vi "Transcriptor LabVIEW to C code Arduino Frontend 2.vi"(11 "vi path":path=path "C:/Users/lubo/Documents/LabView/LabVIEW-Universal-Transcriptor/Test/Examples For Parsing/Blink 4 experimental.vi") -> (3 "transcripted code":string="#include <StandardCplusplus.h>\r\n#include <vector>\r\n#include \"ArduinoBasicFunctions.h\"\nusing namespace std;\r\nstruct UserDefined_StructType{String LuboString;\r\nint NumInsideUserCluter;\r\ndouble Double_insideCluster;\r\n};\r\n\r\n\r\n\nvector<bool> Blink_3_simple_and_correct_one(){\n    UserDefined_StructType totoSomNapisalLenTakSVK wireUID_813_ = {\"LuboJe King\",0,0.000000};\r\n    vector<bool> wireUID_770_;\r\n    vector<bool> wireUID_675_ = {true,true,false};\r\n    /***** BEGIN WhileLoop ********/\n    bool wireUID_529_; //LoopEndRef.Wire\n    do{\n        UserDefined_StructType totoSomNapisalLenTakSVK wireUID_682_ = wireUID_813_;\r\n        UserDefined_StructType totoSomNapisalLenTakSVK wireUID_634_;\r\n        vector<bool> wireUID_729_ = wireUID_675_;\r\n        vector<bool> wireUID_701_;\r\n        int wireUID_426_ = 42;\r\n        double wireUID_569_ = 7.000000;\r\n        int wireUID_540_;\r\n        Delay(wireUID_426_); /* by Translator.vi, VI Path: C:\\Users\\lubo\\Documents\\LabView\\LabVIEW-Universal-Transcriptor\\Test\\Examples For Parsing\\Delay.vi */\r\n        wireUID_529_ = wireUID_569_ > wireUID_540_;\r\n        /***** BEGIN CaseStructure ********/\n        \r\n        UserDefined_StructType totoSomNapisalLenTakSVK wireUID_828_ = wireUID_682_;\r\n        vector<bool> wireUID_820_ = wireUID_729_;\r\n        int wireUID_575_ = -42;\r\n        \r\n        UserDefined_StructType totoSomNapisalLenTakSVK wireUID_670_ = wireUID_682_;\r\n        vector<bool> wireUID_720_ = wireUID_729_;\r\n        int wireUID_953_ = -99; //wires declarations\n        switch(wireUID_529_){\n            case false:\n                \r\n                Delay(wireUID_575_); /* by Translator.vi, VI Path: C:\\Users\\lubo\\Documents\\LabView\\LabVIEW-Universal-Transcriptor\\Test\\Examples For Parsing\\Delay.vi */ /* C code */\n                wireUID_701_ = wireUID_820_;\r\n                wireUID_634_ = wireUID_828_; /* output assgn. */\n            break;\r\n            case true:\n                \r\n                Delay(wireUID_953_); /* by Translator.vi, VI Path: C:\\Users\\lubo\\Documents\\LabView\\LabVIEW-Universal-Transcriptor\\Test\\Examples For Parsing\\Delay.vi */\r\n                Toggle_LED(); /* C code */\n                wireUID_701_ = wireUID_720_;\r\n                wireUID_634_ = wireUID_670_; /* output assgn. */\n            break;\n        }\n        /****** END CaseStructure /* C code */\n        wireUID_770_ = wireUID_701_;\r\n         = wireUID_634_; /* output assgn. */\n    }while(wireUID_529_);\n    /****** END WhileLoop */\r\n    vector<bool> BoolArrayIndicator1 = wireUID_770_;\r\n    \r\n    return BoolArrayIndicator1;\n}\n\nvoid setup(){}\nvoid loop(){\n    Blink_3_simple_and_correct_one();\n}\n")   [LabVIEW 2014]
uses:
  <vilib>/Utility/miscctls.llb/LVPointTypeDef.ctl
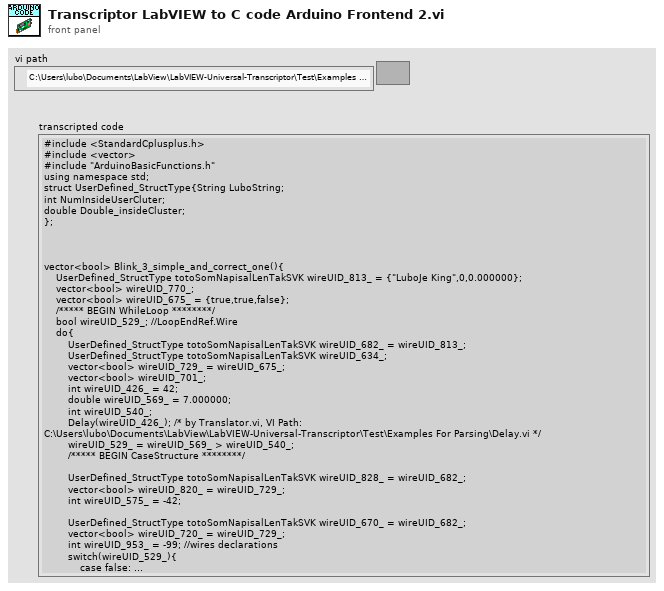
[diagram p1: front panel]
types:
  T1 = typedef "LVPointTypeDef.ctl" = cluster{"Horizontal":i16, "Vertical":i16}
  T2 = typedef "LabVIEW Universal Transcriptor Cluster.ctl" = cluster{"Defines":string[], "Includes":string[], "C code":string, "temp":string[]}
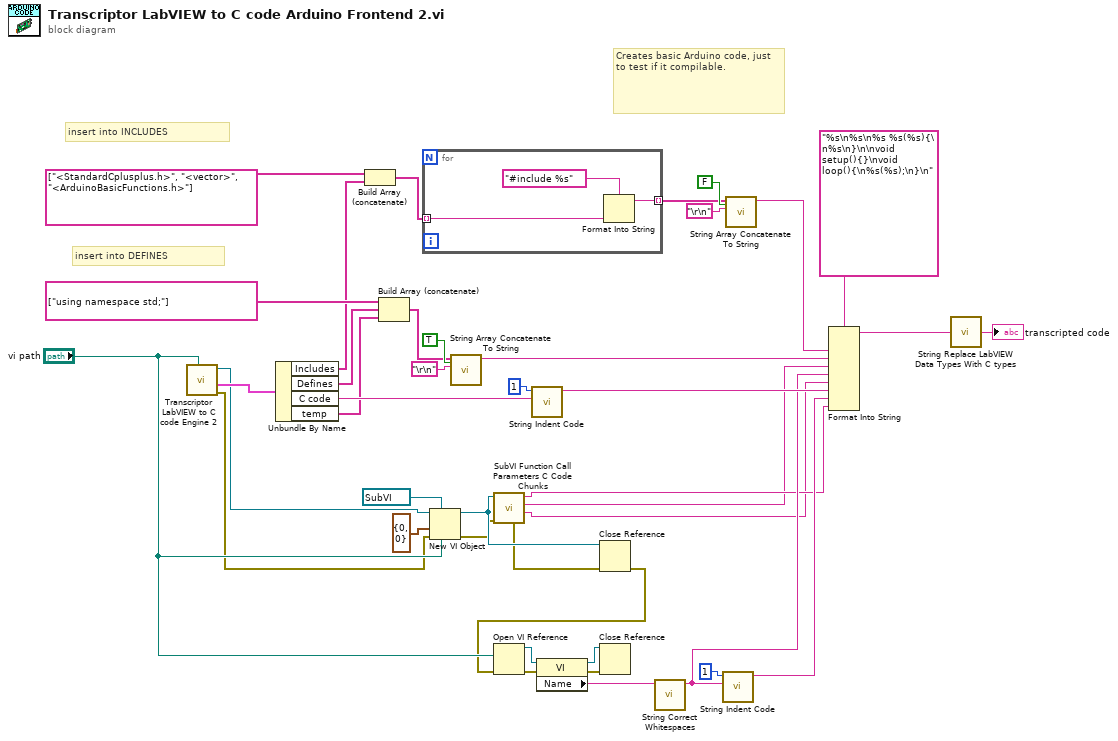
[diagram p0: block diagram]
diagram:
  # "insert into INCLUDES"
  # "insert into DEFINES"
  # "Creates basic Arduino code, just to test if it compilable."
  n1 = call "Transcriptor LabVIEW to C code Engine 2.vi"("vi path"="vi path") -> ("Error Out"=w8:errorcluster, "output cluster"=w41:T2, "Diagram out"=w10:refnum<vi>)  [unwired: 7 in, 1 out]
  n2 = Unbundle By Name(w41) -> ("Includes"=w18:string[], "Defines"=w21:string[], "C code"=w29:string, "temp"=w1:string[])
  n3 = Build Array (concatenate)(string[] ["<StandardCplusplus.h>", "<vector>", "<ArduinoBasicFunctions.h>"], w18) -> (w17:string[])
  n4 = Build Array (concatenate)(string[] ["using namespace std;"], w21, w1) -> (w20:string[])
  n5 = for {
    tunnel: w17 -> [w43] mode=indexing
    tunnel: [w42] -> w33 mode=indexing
    n6 = Format Into String(format string="#include %s", w43) -> (resulting string=w42:string)  [unwired: 2 in, 1 out]
  }
  n7 = New VI Object(vi object class=refnum<vi> refnum ("Diagram out"), owner refnum=w10, position/next to=T1 {"Horizontal"=0, "Vertical"=0} ("location"), 6:"vi path", 8:w8) -> (object refnum=w7:refnum<vi>, 0:w4:errorcluster)  [unwired: 3 in]
  n8 = call "String Array Concatenate To String.vi"("insert last delimiter?"=TRUE, "Delimiter char"="\r\n", "Array String In"=w20) -> ("String"=w38:string)  [unwired: 8 in]
  n9 = call "SubVI Function Call Parameters C Code Chunks.vi"("Error In"=w4, "SubVI Refnum"=w7) -> ("SubVI func. params  declaration"=w13:string, "return datatype"=w14:string, "SubVI func. call params"=w15:string, "Error Out"=w3:errorcluster)  [unwired: 5 in, 1 out]
  n10 = call "String Indent Code.vi"("complete code"=w29, "actual nested level"=1) -> ("indented code"=w28:string)  [unwired: 9 in]
  n11 = Close Reference(reference=w7, error in (no error)=w3) -> (error out=w2:errorcluster)
  n12 = Open VI Reference(vi path="vi path", error in (no error)=w2) -> (vi reference=w11:refnum<vi>, error out=w32:errorcluster)  [unwired: 4 in]
  n13 = property class="VI"(reference=w11, error in=w32) -> (reference out=w12:refnum<vi>, error out=w30:errorcluster, "Name"=w31:string)
  n14 = Close Reference(reference=w12, error in (no error)=w30) -> ()  [unwired: 1 out]
  n15 = call "String Correct Whitespaces.vi"("String in"=w31) -> ("String out"=w25:string)  [unwired: 10 in]
  n16 = call "String Indent Code.vi"("complete code"=w25, "actual nested level"=1) -> ("indented code"=w24:string)  [unwired: 9 in]
  n17 = call "String Array Concatenate To String.vi"("insert last delimiter?"=FALSE, "Delimiter char"="\r\n", "Array String In"=w33) -> ("String"=w34:string)  [unwired: 8 in]
  n18 = Format Into String(format string="%s\n%s\n%s %s(%s){\n%s\n}\n\nvoid setup(){}\nvoid loop(){\n%s(%s);\n}\n", w34, w38, w14, w25, w13, w28, w24, w15) -> (resulting string=w23:string)  [unwired: 2 in, 1 out]
  n19 = call "String Replace LabVIEW Data Types With C types.vi"("C code"=w23) -> ("C code, replaced datatypes"=→"transcripted code":string)
